vi "dsfsdfsd_Write Array.vi"(8 "error in (no error)":errorcluster, 10 "Array":cluster{"Numeric":dbl, "String":string}[](array[cluster]), 11 "dsfsdfsd in":refnum<class "dsfsdfsd.lvclass">) -> (0 "error out":errorcluster, 3 "dsfsdfsd out":refnum<class "dsfsdfsd.lvclass">)   [LabVIEW 2013, in "dsfsdfsd.lvclass"]
uses:
  dsfsdfsd.lvclass
  dsfsdfsd.lvclass/dsfsdfsd.ctl
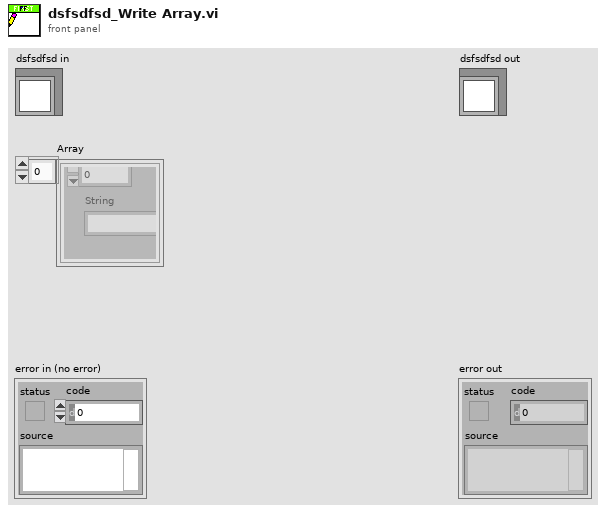
[diagram p1: front panel]
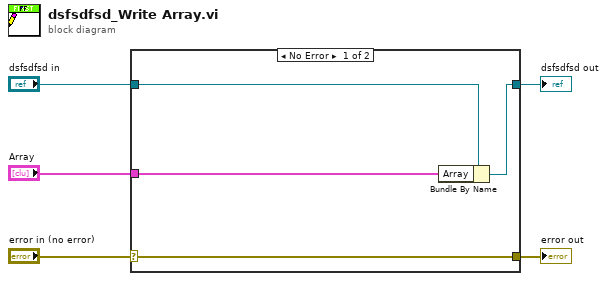
[diagram p0: block diagram]
diagram:
  n1 = case shown="No Error" "error in (no error)" {
    selector: "error in (no error)" -> [w9 w10]
    tunnel: [w9 w10] -> w4
    tunnel: [w7 w11] -> w2
    tunnel: "dsfsdfsd in" -> [w8 w11]
    tunnel: "Array" -> [w6 _]
    frame No Error {
      n2 = Bundle By Name(cluster=w8, "Array"=w6) -> (w7:refnum<class "dsfsdfsd.lvclass">)
    }
    frame Error {
    }
  }
  "error out" <- w4
  "dsfsdfsd out" <- w2
